vi "Graph Supersize v10.6.2.vi"() -> ()   [LabVIEW 2010]
uses:
  <vilib>/Utility/miscctls.llb/LVPointTypeDef.ctl
panel:
  in  "SpectrumAxis":string
  in  "AutoClose":bool
  out "Image":dbl[][](graph)
  in  "Exit":bool
  out "Spectrum":cluster{dbl[], dbl[]}[](graph)
  in  "Image Mode":bool caption="Image Mode?"
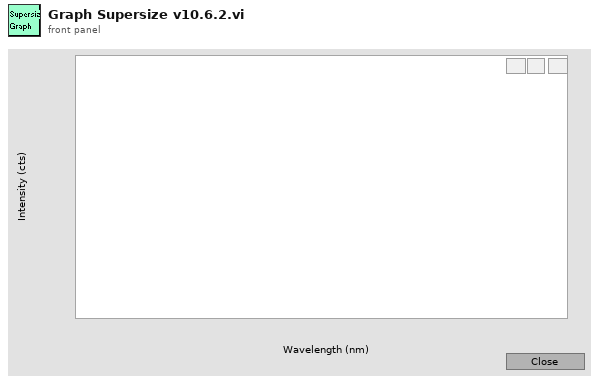
[diagram p1: front panel]
types:
  T1 = enum16{"No Scaling", "Scale All Objects", "Scale Single Object"}
  T2 = typedef "LVPointTypeDef.ctl" = cluster{"Horizontal":i16, "Vertical":i16}
  T3 = enum16{"fire", "rainbow", "gray", "inverse gray", "ice", "original"}
  T4 = enum32{"invalid app kind", "Development System", "Run Time System", "Student Edition", "Embedded LabVIEW", "Evaluation", "Custom"}
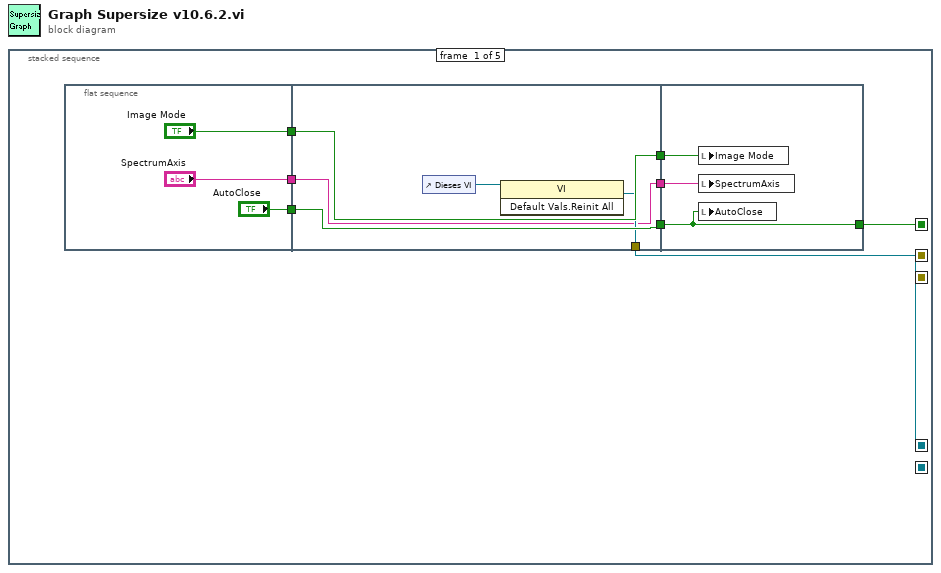
[diagram p0: block diagram]
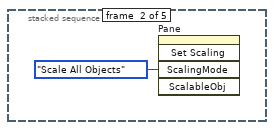
[diagram p2: hidden frame]
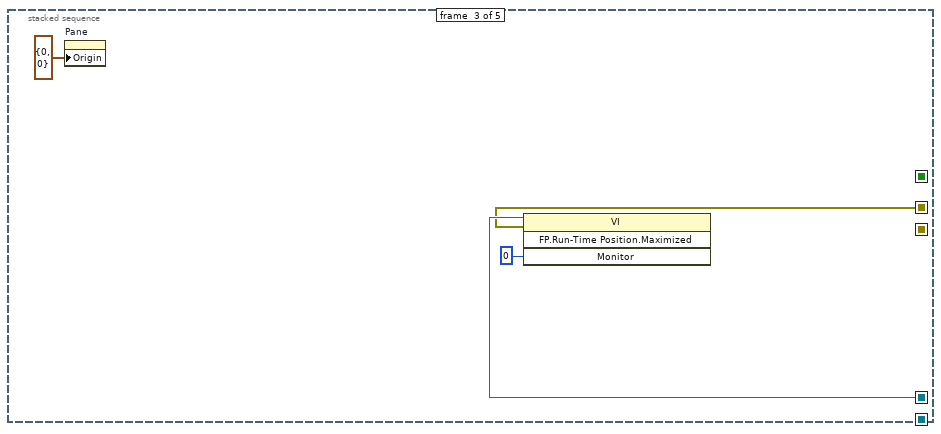
[diagram p3: hidden frame]
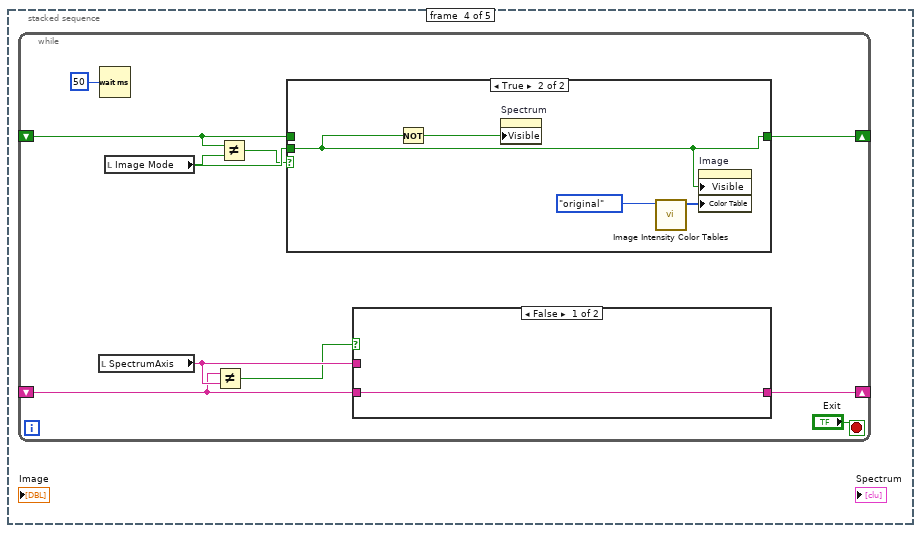
[diagram p4: hidden frame]
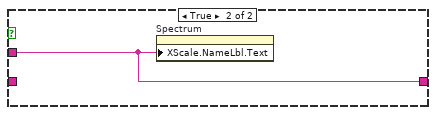
[diagram p5: hidden frame]
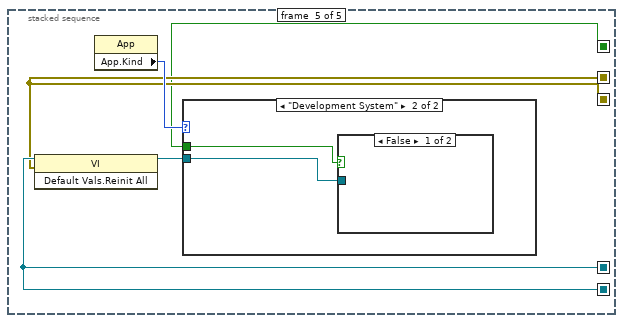
[diagram p7: hidden frame]
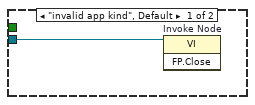
[diagram p8: hidden frame]
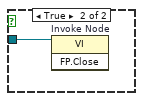
[diagram p9: hidden frame]
diagram:
  n1 = stacked-sequence {
    seq-local: [w5 _ _ _ _] -> [_ _ w24 _ w46]
    seq-local: [w4 _ _ _ _] -> [_ _ w23 _ w45]
    seq-local: [_ _ _ _ w46] -> [_ _ _ _ _]
    seq-local: [_ _ _ _ w45] -> [_ _ _ _ _]
    seq-local: [w1 _ _ _ _] -> [_ _ _ _ w44]
    frame #0 {
      n2 = flat-sequence {
        tunnel: ["Image Mode"] -> w9
        tunnel: ["AutoClose"] -> w8
        tunnel: ["SpectrumAxis"] -> w2
        tunnel: [w17] -> w7
        tunnel: w9 -> [w17]
        tunnel: [w16] -> w6
        tunnel: w8 -> [w16]
        tunnel: [w15] -> w5
        tunnel: [w14] -> w4
        tunnel: [w13] -> w3
        tunnel: w2 -> [w13]
        tunnel: w7 -> [w21]
        tunnel: w6 -> [w19]
        tunnel: w3 -> [w20]
        tunnel: [w19] -> w1
        frame #0 {
        }
        frame #1 {
          n3 = control-ref of="Dieses VI"() -> (w18:refnum<vi>)
          n4 = invoke class="VI" method="Default Vals.Reinit All"(reference=w18) -> (reference out=w15:refnum<vi>, error out=w14:errorcluster)  [unwired: 2 in, 1 out]
        }
        frame #2 {
          n5 = local write "Image Mode"(w21) -> ()
          n6 = local write "SpectrumAxis"(w20) -> ()
          n7 = local write "AutoClose"(w19) -> ()
        }
      }
    }
    frame #1 {
      n8 = invoke on="Pane" class="Pane" method="Set Scaling"("ScalingMode"=T1."Scale All Objects" ("Scaling Mode")) -> ()  [unwired: 4 in, 5 out]
    }
    frame #2 {
      n9 = property on="Pane" class="Pane"("Origin"=T2 {"Horizontal"=0, "Vertical"=0}) -> ()  [unwired: 2 in, 2 out]
      n10 = invoke class="VI" method="FP.Run-Time Position.Maximized"(reference=w24, error in=w23, "Monitor"=i16 0) -> ()  [unwired: 1 in, 4 out]
    }
    frame #3 {
      n11 = while {
        shift-right: [w32] -> _
        shift-left: _ -> [w31]
        shift-right: [w28] -> _
        shift-left: _ -> [w29]
        stop <- "Exit" stop-if-true
        n12 = local read "SpectrumAxis"() -> (w30:string)
        n13 = Wait (ms)(milliseconds to wait=50) -> ()  [unwired: 1 out]
        n14 = local read "Image Mode"() -> (w34:bool)
        n15 = Not Equal?(x=w29, y=w30) -> (x != y?=w27:bool)
        n16 = Not Equal?(x=w31, y=w34) -> (x != y?=w33:bool)
        n17 = case shown="True" w33 {
          tunnel: w34 -> [_ w40]
          tunnel: [w39 w40] -> w32
          tunnel: w31 -> [w39 _]
          frame False {
          }
          frame True {
            n18 = Not(x=w40) -> (.not. x?=w41:bool)
            n19 = property on="Spectrum" class="XYGraph (strict)"("Visible"=w41) -> ()  [unwired: 2 in, 2 out]
            n20 = call "Image Intensity Color Tables.vi"("Map Selector"=T3."original") -> ("Color Map Array"=w42:u32[])  [unwired: 10 in]
            n21 = property on="Image" class="IntGraph (strict)"("Visible"=w40, "Color Table"=w42) -> ()  [unwired: 2 in, 2 out]
          }
        }
        n22 = case shown="False" w27 {
          tunnel: w30 -> [_ w38]
          tunnel: [w37 w38] -> w28
          tunnel: w29 -> [w37 _]
          frame False {
          }
          frame True {
            n23 = property on="Spectrum" class="XYGraph (strict)"("XScale.NameLbl.Text"=w38) -> ()  [unwired: 2 in, 2 out]
          }
        }
      }
    }
    frame #4 {
      n24 = invoke class="VI" method="Default Vals.Reinit All"(reference=w46, error in=w45) -> (reference out=w47:refnum<vi>)  [unwired: 1 in, 2 out]
      n25 = property class="App"() -> ("App.Kind"=w48:T4)  [unwired: 2 in, 2 out]
      n26 = case shown="\"Development System\"" w48 {
        tunnel: w47 -> [w49 w51]
        tunnel: w44 -> [_ w50]
        frame "invalid app kind", Default {
          n27 = invoke on="Invoke Node" class="VI" method="FP.Close"(reference=w49) -> ()  [unwired: 2 in, 3 out]
        }
        frame "Development System" {
          n28 = case shown="False" w50 {
            tunnel: w51 -> [_ w52]
            frame False {
            }
            frame True {
              n29 = invoke on="Invoke Node" class="VI" method="FP.Close"(reference=w52) -> ()  [unwired: 2 in, 3 out]
            }
          }
        }
      }
    }
  }
